vi "getFilterFrequencies.vi"(8 "error in (no error)":errorcluster, 11 "pHandle":u32) -> (0 "error out":errorcluster, 1 "cutoffAccel":sgl, 2 "cutoffGyro":sgl, 3 "gyroAccelsSampling":sgl, 4 "cutoffMagneto":sgl, 5 "mainLoopFrequency":sgl, 6 "return type":i32)   [LabVIEW 2011, in "sbgLabView.lvlib"]
uses:
  sbgLabView.lvlib
  sbgMatLab.dll
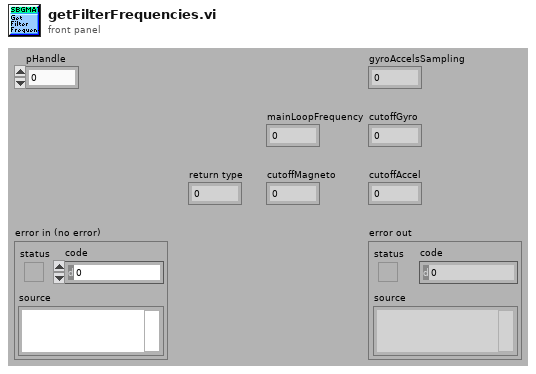
[diagram p1: front panel]
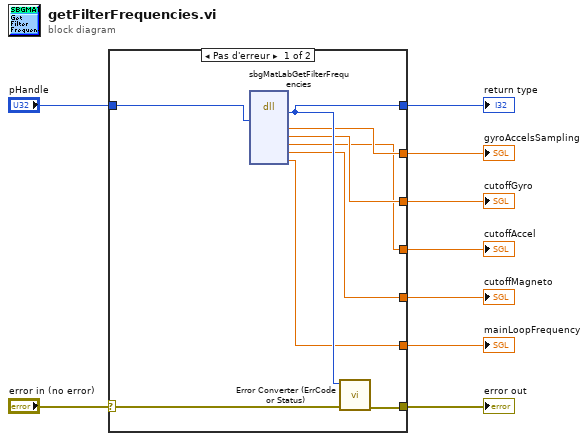
[diagram p0: block diagram]
diagram:
  n1 = case shown="Pas d'erreur" "error in (no error)" {
    selector: "error in (no error)" -> [w11 w19]
    tunnel: [w10 w19] -> w8
    tunnel: [w18 _] -> w7
    tunnel: "pHandle" -> [w17 _]
    tunnel: [w16 _] -> w5
    tunnel: [w15 _] -> w4
    tunnel: [w14 _] -> w3
    tunnel: [w13 _] -> w2
    tunnel: [w12 _] -> w1
    frame No Error {
      n2 = dll-call lib="C:/SBG-Systems/remote/projects/software/projects/labviewExample/sbgLabView/sbgMatLab.*" fn="sbgMatLabGetFilterFrequencies"("pHandle"=w17) -> ("type de retour"=w18:i32, "pGyroAccelsSampling"=w16:sgl, "pCutoffGyro"=w15:sgl, "pCutoffAccel"=w14:sgl, "pCutoffMagneto"=w13:sgl, "pMainLoopFrequency"=w12:sgl)  [unwired: 9 in, 2 out]
      n3 = call "Error Converter (ErrCode or Status).vi"("error in (no error)"=w11, "error code"=w18) -> ("error out"=w10:errorcluster)  [unwired: 9 in]
    }
    frame Error {
    }
  }
  "return type" <- w7
  "gyroAccelsSampling" <- w5
  "cutoffGyro" <- w4
  "cutoffAccel" <- w3
  "cutoffMagneto" <- w2
  "mainLoopFrequency" <- w1
  "error out" <- w8
